vi "PicoScope6000aGetStreamingTriggerInfo.vi"(2 "enabled array":i16[](array[numeric])=[1, 0, 0, 0, 0, 0, 0, 0, 0, 0], 5 "No of C Strutures":u64=1, 7 "C Struture define":T2={"Channel"=0, "Down-Sample Mode"=2147483648, "PICO_DATA_TYPE"=enum."PICO_INT16_T", "Samples"=1000000, "bufferIndex"=0, "startIndex"=0, "overflow"=0} {"overflow" step=1; "Down-Sample Mode" items=["None"=2147483648, "Aggregate"=1, "Decimate"=2, "Average"=4]; "Channel" items=["Channel A"=0, "Channel B"=1, "Channel C"=2, "Channel D"=3, "Channel E"=4, "Channel F"=5, "Channel G"=6, "Channel H"=7, "Port 0"=128, "Port 1"=129, "Trigger AUX"=1001]; "startIndex" step=1}, 9 "C Array for Struture Data In":u16[][](array[numeric]), 11 "error in":errorcluster) -> (8 "C Array for Struture Data Out":u16[][](array[numeric]), 10 "Array of Clusters":T1(array[cluster]) {"overflow" step=1; "Down-Sample Mode" items=["None"=2147483648, "Aggregate"=1, "Decimate"=2, "Average"=4]; "Channel" items=["Channel A"=0, "Channel B"=1, "Channel C"=2, "Channel D"=3, "Channel E"=4, "Channel F"=5, "Channel G"=6, "Channel H"=7, "Port 0"=128, "Port 1"=129, "Trigger AUX"=1001]; "startIndex" step=1}, 15 "error out":errorcluster)   [LabVIEW 2016]
doc: "This VIcan be used for one or two functions-\n-Converts a cluster defined for C struture defined to 2D array to pass to a C shared library function.\n-Converts a 2D array returned from a C shared library functionas an array of clusters representing the C struture"
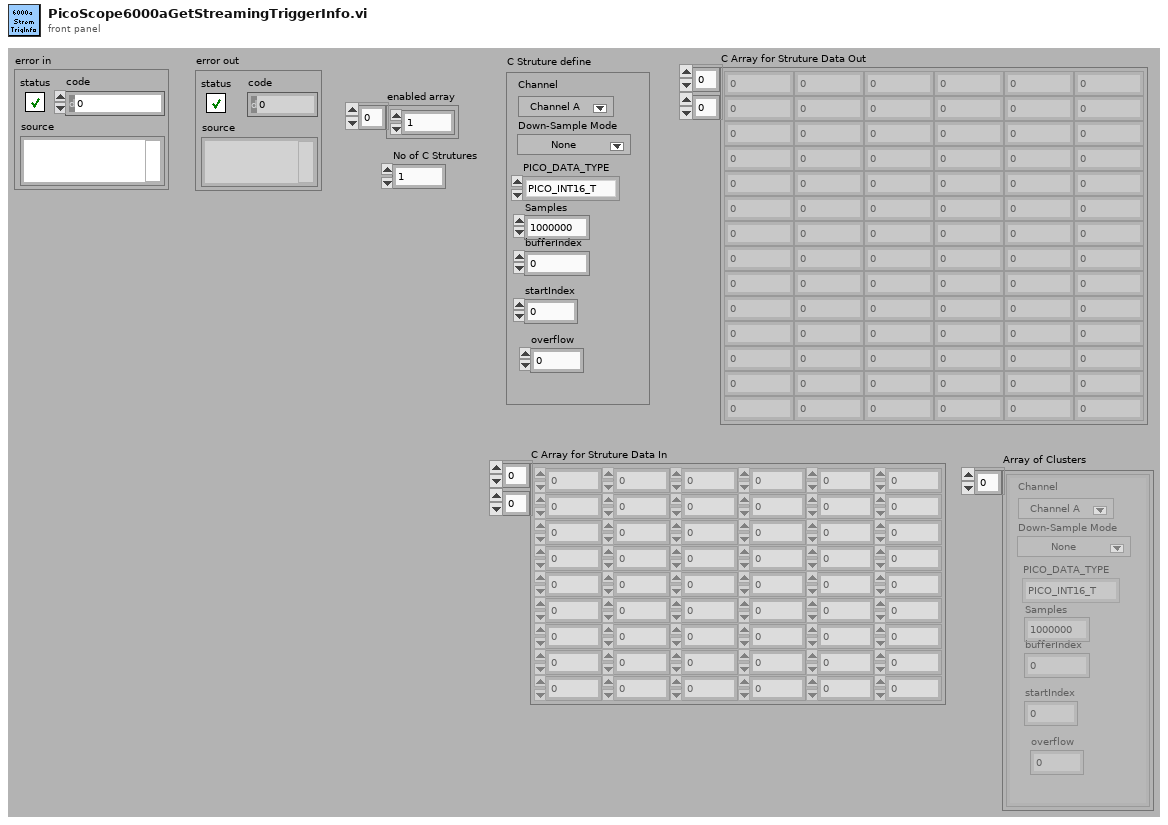
[diagram p1: front panel]
types:
  T1 = cluster{"Channel":u32, "Down-Sample Mode":u32, "PICO_DATA_TYPE":enum32{"PICO_INT8_T", "PICO_INT16_T", "PICO_INT32_T", "PICO_UINT32_T", "PICO_INT64_T", ""}, "Samples":i32, "bufferIndex":u64, "startIndex":i32, "overflow":i16}[]
  T2 = cluster{"Channel":u32, "Down-Sample Mode":u32, "PICO_DATA_TYPE":enum32{"PICO_INT8_T", "PICO_INT16_T", "PICO_INT32_T", "PICO_UINT32_T", "PICO_INT64_T", ""}, "Samples":i32, "bufferIndex":u64, "startIndex":i32, "overflow":i16}
  T3 = enum32{"PICO_INT8_T", "PICO_INT16_T", "PICO_INT32_T", "PICO_UINT32_T", "PICO_INT64_T", ""}
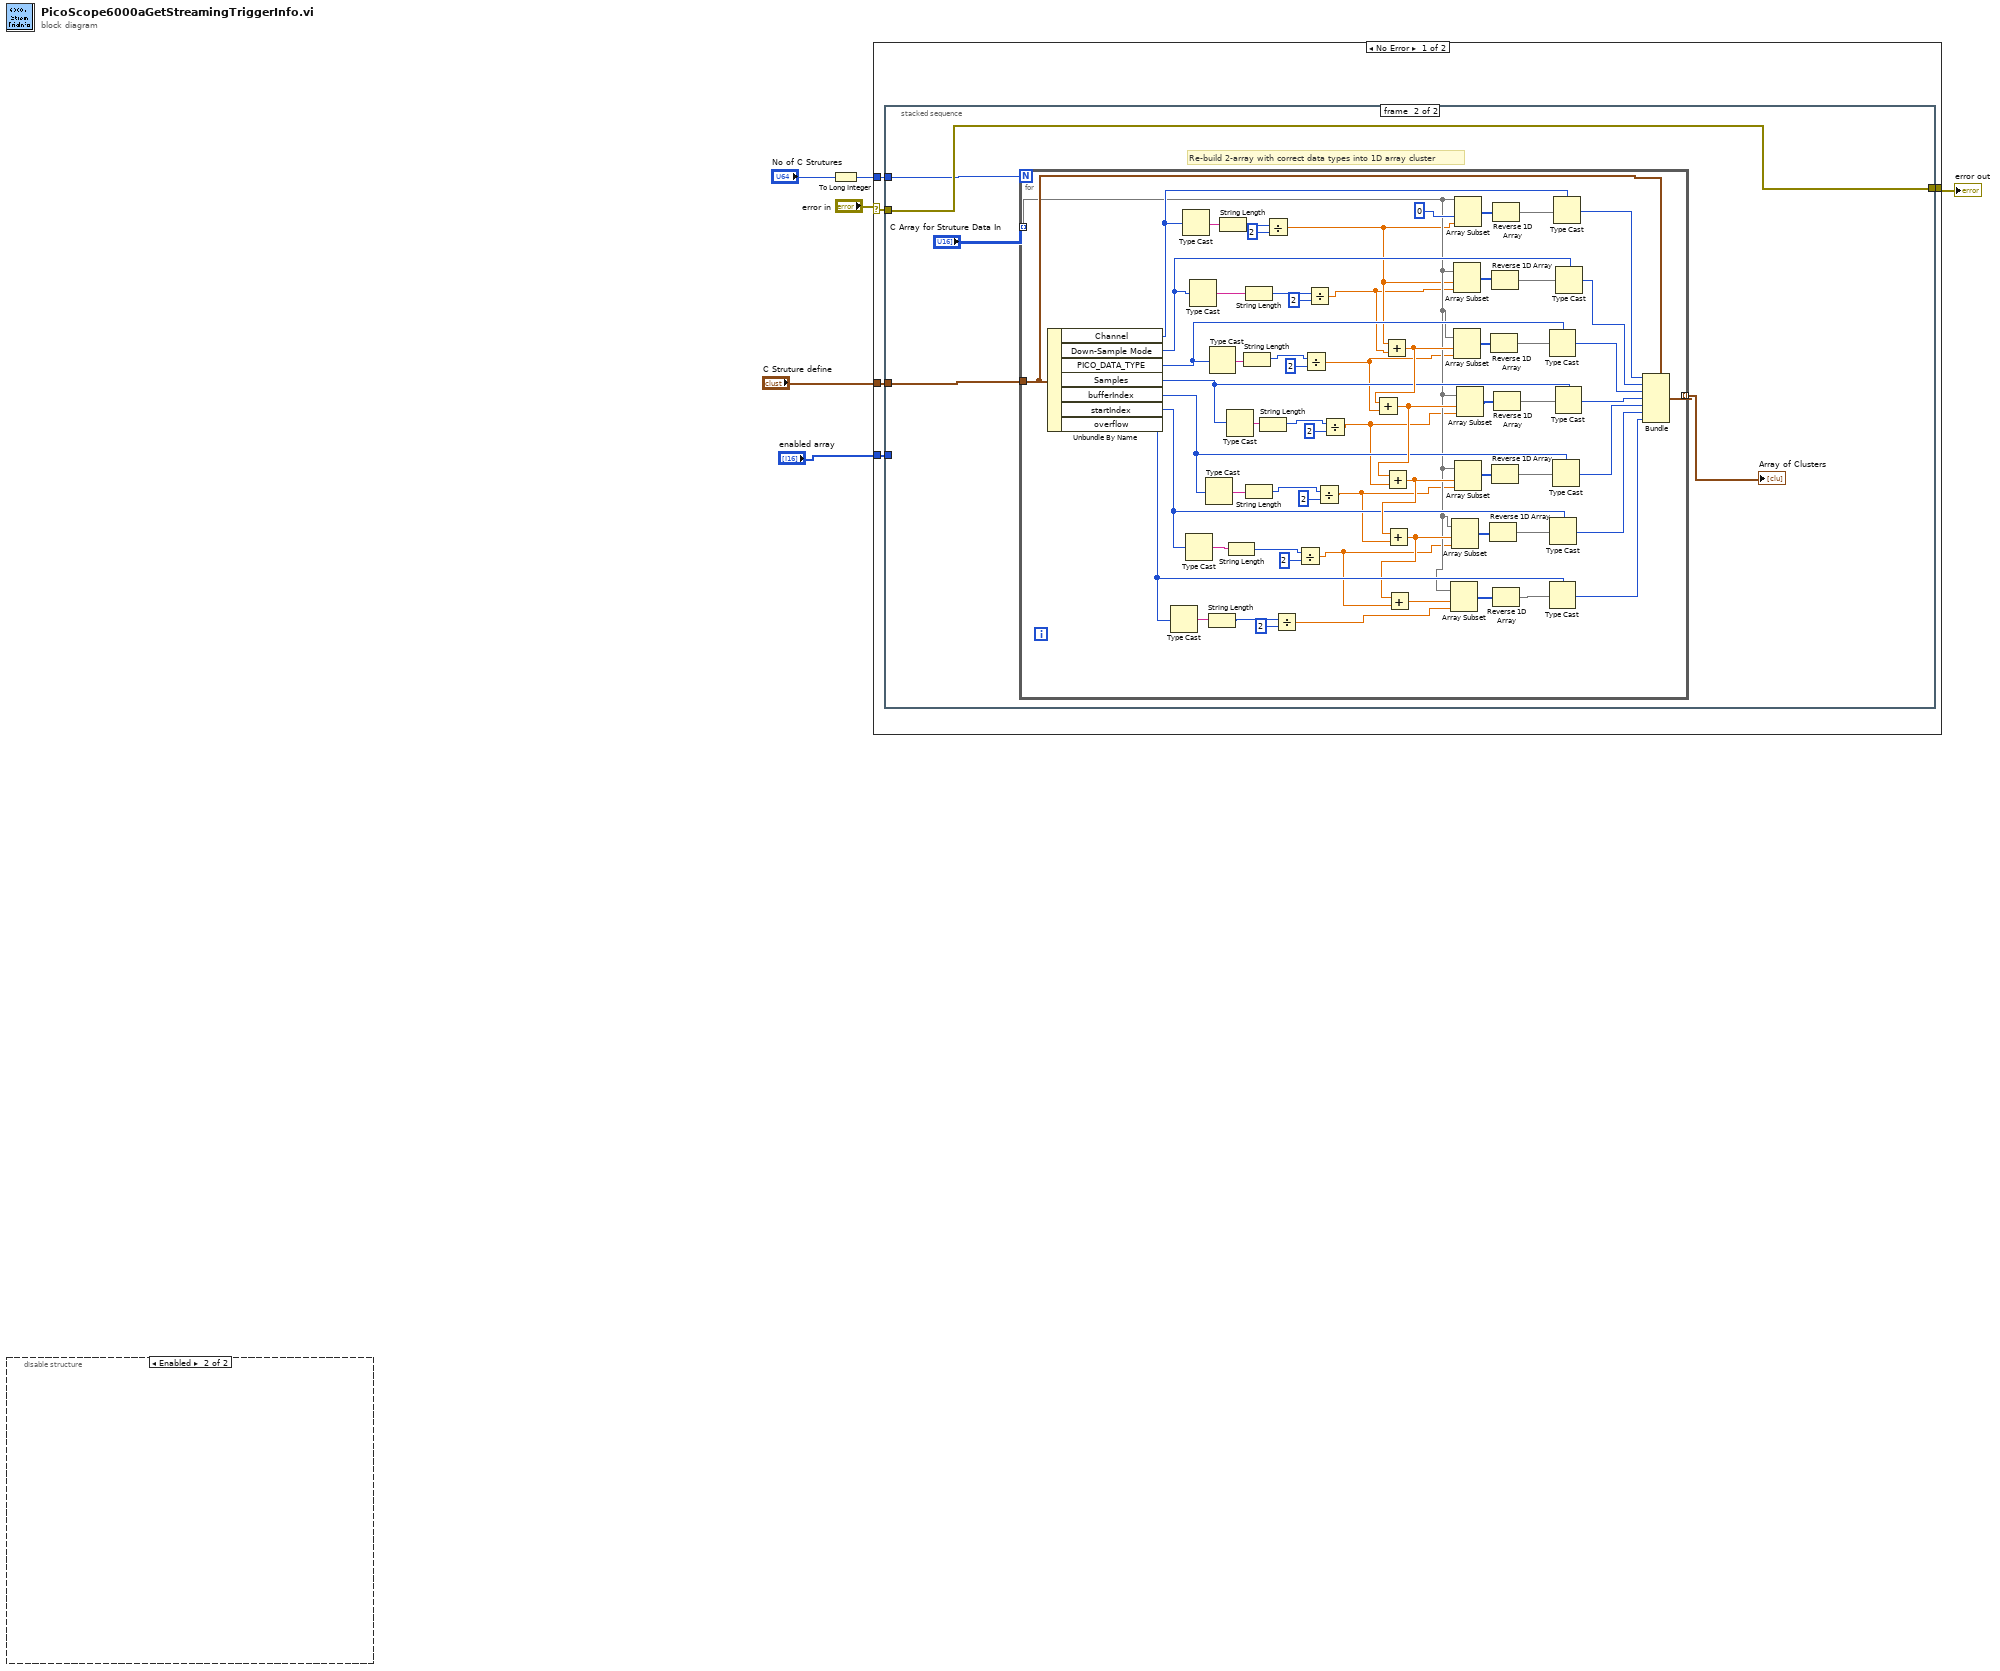
[diagram p0: block diagram]
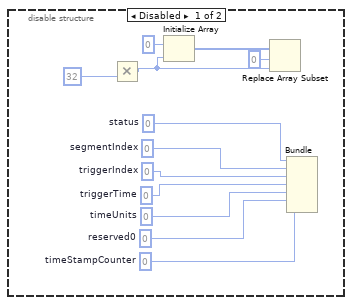
[diagram p2: hidden frame]
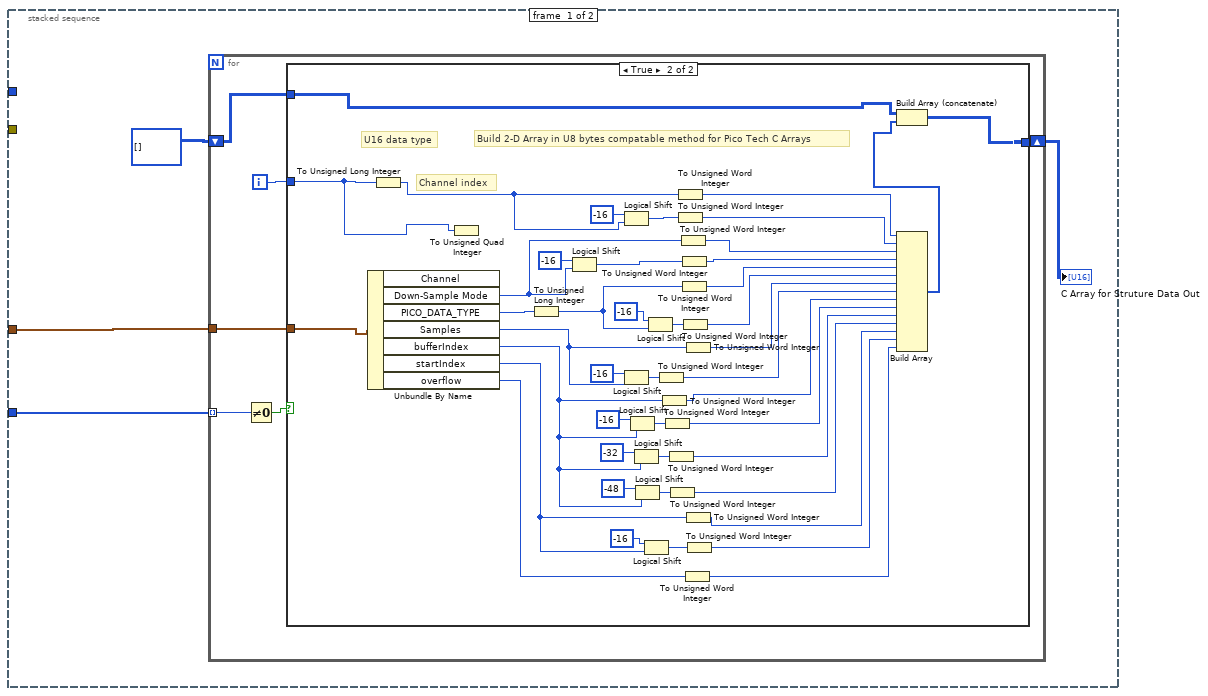
[diagram p3: hidden frame]
diagram:
  n1 = disable-structure shown="Enabled" {
    frame Disabled {
      w14 = u64 0  # timeStampCounter
      w12 = i16 0  # reserved0
      w13 = i16 0  # timeUnits
      w15 = i64 0  # triggerTime
      w16 = u32 0  # triggerIndex
      w17 = u32 0  # segmentIndex
      w18 = u32 0  # status
      n2 = Multiply(y=u32 32) -> (x*y=w10:u32)  [unwired: 1 in]
      n3 = Initialize Array(u8 0 ("element"), w10) -> (w11:u8[])
      n4 = Replace Array Subset(array=w11, new element=w10, index=0) -> ()  [unwired: 1 out]
      n5 = Bundle("status"=w18, "segmentIndex"=w17, "triggerIndex"=w16, "triggerTime"=w15, "timeUnits"=w13, "reserved0"=w12, "timeStampCounter"=w14) -> ()  [unwired: 1 in, 1 out]
    }
    frame Enabled {
    }
  }
  n6 = To Long Integer(number="No of C Strutures") -> (32bit integer=w1:i32)
  n7 = case shown="No Error" "error in" {
    selector: "error in" -> [w23 w149]
    tunnel: [w22 w149] -> w5
    tunnel: w1 -> [w21 _]
    tunnel: "C Struture define" -> [w20 _]
    tunnel: "enabled array" -> [w19 _]
    frame No Error {
      n8 = stacked-sequence {
        tunnel: w23 -> [_ w83]
        tunnel: [_ w83] -> w22
        tunnel: w21 -> [_ w82]
        tunnel: w20 -> [w26 w81]
        tunnel: w19 -> [w25 _]
        frame #0 {
          # "Build 2-D Array in U8 bytes compatable method for Pico Tech C Arrays"
          n9 = for {
            tunnel: w26 -> [w33]
            tunnel: w25 -> [w32] mode=indexing
            shift-right: [w28] -> w27
            shift-left: u16[][] [] -> [w29]
            i -> [w30]
            n10 = Not Equal To 0?(x=w32) -> (x != 0?=w31:bool)
            n11 = case shown="True" w31 {
              tunnel: w33 -> [_ w78]
              tunnel: w30 -> [_ w36]
              tunnel: w29 -> [w34 w39]
              tunnel: [w34 w37] -> w28
              frame False {
              }
              frame True {
                # "Channel index"
                # "U16 data type"
                n12 = Unbundle By Name(w78) -> ("Down-Sample Mode"=w62:u32, "PICO_DATA_TYPE"=w61:T3, "Samples"=w59:i32, "bufferIndex"=w35:u64, "startIndex"=w45:i32, "overflow"=w44:i16)  [unwired: 1 out]
                n13 = To Unsigned Long Integer(number=w36) -> (unsigned 32bit integer=w40:u32)
                n14 = To Unsigned Quad Integer(1:w36) -> ()  [unwired: 1 out]
                n15 = To Unsigned Long Integer(number=w61) -> (unsigned 32bit integer=w60:u32)
                n16 = Logical Shift(y=i16 -16, x=w62) -> (x << y=w75:u32)
                n17 = Logical Shift(y=i16 -16, x=w40) -> (x << y=w76:u32)
                n18 = Logical Shift(y=i16 -16, x=w59) -> (x << y=w71:i32)
                n19 = Logical Shift(y=i16 -16, x=w35) -> (x << y=w55:u64)
                n20 = Logical Shift(y=i16 -32, x=w35) -> (x << y=w54:u64)
                n21 = Logical Shift(y=i16 -48, x=w35) -> (x << y=w52:u64)
                n22 = Logical Shift(y=i16 -16, x=w45) -> (x << y=w46:i32)
                n23 = Logical Shift(y=i16 -16, x=w60) -> (x << y=w72:u32)
                n24 = To Unsigned Word Integer(number=w71) -> (unsigned 16bit integer=w51:u16)
                n25 = To Unsigned Word Integer(number=w35) -> (unsigned 16bit integer=w50:u16)
                n26 = To Unsigned Word Integer(number=w55) -> (unsigned 16bit integer=w49:u16)
                n27 = To Unsigned Word Integer(number=w54) -> (unsigned 16bit integer=w48:u16)
                n28 = To Unsigned Word Integer(number=w52) -> (unsigned 16bit integer=w47:u16)
                n29 = To Unsigned Word Integer(number=w40) -> (unsigned 16bit integer=w69:u16)
                n30 = To Unsigned Word Integer(number=w76) -> (unsigned 16bit integer=w68:u16)
                n31 = To Unsigned Word Integer(number=w62) -> (unsigned 16bit integer=w67:u16)
                n32 = To Unsigned Word Integer(number=w75) -> (unsigned 16bit integer=w66:u16)
                n33 = To Unsigned Word Integer(number=w60) -> (unsigned 16bit integer=w65:u16)
                n34 = To Unsigned Word Integer(number=w72) -> (unsigned 16bit integer=w64:u16)
                n35 = To Unsigned Word Integer(number=w44) -> (unsigned 16bit integer=w41:u16)
                n36 = To Unsigned Word Integer(number=w59) -> (unsigned 16bit integer=w63:u16)
                n37 = To Unsigned Word Integer(number=w45) -> (unsigned 16bit integer=w43:u16)
                n38 = To Unsigned Word Integer(number=w46) -> (unsigned 16bit integer=w42:u16)
                n39 = Build Array(w69, w68, w67, w66, w65, w64, w63, w51, w50, w49, w48, w47, w43, w42, w41) -> (w38:u16[])
                n40 = Build Array (concatenate)(w39, w38) -> (w37:u16[][])
              }
            }
          }
          "C Array for Struture Data Out" <- w27
        }
        frame #1 {
          # "Re-build 2-array with correct data types into 1D array cluster"
          n41 = for {
            N: w82 -> [_]
            tunnel: "C Array for Struture Data In" -> [w106] mode=indexing
            tunnel: [w145] -> w80 mode=indexing
            tunnel: w81 -> [w107]
            n42 = Unbundle By Name(w107) -> ("Channel"=w119:u32, "Down-Sample Mode"=w118:u32, "PICO_DATA_TYPE"=w114:T3, "Samples"=w115:i32, "bufferIndex"=w116:u64, "startIndex"=w110:i32, "overflow"=w117:i16)
            n43 = Type Cast(x=w117) -> (*(type *) &x=w124:string)  [unwired: 1 in]
            n44 = Type Cast(x=w119) -> (*(type *) &x=w105:string)  [unwired: 1 in]
            n45 = Type Cast(x=w110) -> (*(type *) &x=w128:string)  [unwired: 1 in]
            n46 = Type Cast(x=w118) -> (*(type *) &x=w132:string)  [unwired: 1 in]
            n47 = Type Cast(x=w116) -> (*(type *) &x=w129:string)  [unwired: 1 in]
            n48 = String Length(string=w124) -> (length=w95:i32)
            n49 = Type Cast(x=w114) -> (*(type *) &x=w131:string)  [unwired: 1 in]
            n50 = String Length(string=w105) -> (length=w104:i32)
            n51 = Type Cast(x=w115) -> (*(type *) &x=w130:string)  [unwired: 1 in]
            n52 = String Length(string=w128) -> (length=w86:i32)
            n53 = String Length(string=w131) -> (length=w92:i32)
            n54 = String Length(string=w132) -> (length=w93:i32)
            n55 = String Length(string=w129) -> (length=w88:i32)
            n56 = String Length(string=w130) -> (length=w89:i32)
            n57 = Divide(x=w104, y=2) -> (x/y=w102:dbl)
            n58 = Divide(x=w95, y=2) -> (x/y=w85:dbl)
            n59 = Divide(x=w86, y=2) -> (x/y=w84:dbl)
            n60 = Divide(x=w92, y=2) -> (x/y=w91:dbl)
            n61 = Divide(x=w93, y=2) -> (x/y=w94:dbl)
            n62 = Divide(x=w88, y=2) -> (x/y=w87:dbl)
            n63 = Divide(x=w89, y=2) -> (x/y=w90:dbl)
            n64 = Add(x=w102, y=w94) -> (x+y=w121:dbl)
            n65 = Add(x=w121, y=w91) -> (x+y=w127:dbl)
            n66 = Add(x=w127, y=w90) -> (x+y=w126:dbl)
            n67 = Add(x=w126, y=w87) -> (x+y=w113:dbl)
            n68 = Add(x=w113, y=w84) -> (x+y=w123:dbl)
            n69 = Array Subset(array=w106, index=w123, length=w85) -> (w122:u16[])
            n70 = Array Subset(array=w106, index=w113, length=w84) -> (w112:u16[])
            n71 = Array Subset(array=w106, index=w102, length=w94) -> (w144:u16[])
            n72 = Array Subset(array=w106, index=w121, length=w91) -> (w139:u16[])
            n73 = Array Subset(array=w106, index=0, length=w102) -> (w142:u16[])
            n74 = Array Subset(array=w106, index=w126, length=w87) -> (w136:u16[])
            n75 = Array Subset(array=w106, index=w127, length=w90) -> (w138:u16[])
            n76 = Reverse 1D Array(array=w112) -> (reversed array=w111:u16[])
            n77 = Reverse 1D Array(array=w139) -> (reversed array=w140:u16[])
            n78 = Reverse 1D Array(array=w144) -> (reversed array=w143:u16[])
            n79 = Reverse 1D Array(array=w136) -> (reversed array=w135:u16[])
            n80 = Reverse 1D Array(array=w142) -> (reversed array=w141:u16[])
            n81 = Reverse 1D Array(array=w122) -> (reversed array=w134:u16[])
            n82 = Reverse 1D Array(array=w138) -> (reversed array=w137:u16[])
            n83 = Type Cast(type=w114, x=w140) -> (*(type *) &x=w148:T3)
            n84 = Type Cast(type=w117, x=w134) -> (*(type *) &x=w108:i16)
            n85 = Type Cast(type=w110, x=w111) -> (*(type *) &x=w109:i32)
            n86 = Type Cast(type=w116, x=w135) -> (*(type *) &x=w146:u64)
            n87 = Type Cast(type=w119, x=w141) -> (*(type *) &x=w120:u32)
            n88 = Type Cast(type=w115, x=w137) -> (*(type *) &x=w147:i32)
            n89 = Type Cast(type=w118, x=w143) -> (*(type *) &x=w133:u32)
            n90 = Bundle(cluster=w107, "Channel"=w120, "Down-Sample Mode"=w133, "PICO_DATA_TYPE"=w148, "Samples"=w147, "bufferIndex"=w146, "startIndex"=w109, "overflow"=w108) -> (w145:T2)
          }
          "Array of Clusters" <- w80
        }
      }
    }
    frame Error {
    }
  }
  "error out" <- w5
